vi "AlliGator Python Plugin Plot Data Type.vi"(8 "error in (no error)":errorcluster, 11 "Function Name":string) -> (0 "error out":errorcluster, 3 "Type of Plot Data":T1)   [LabVIEW 2021, in "AlliGator Python Plugins.lvlib"]
doc: "Looks at the python function name to figure out whether it acts on \"All Plots\" or \"Selected Plots\"."
uses:
  AlliGator Python Plugins.lvlib
  AlliGator Type of Plot Data.ctl
panel:
  # "see the AlliGator License on the block diagram (Ctrl+E or Window:Show Block Diagram)"
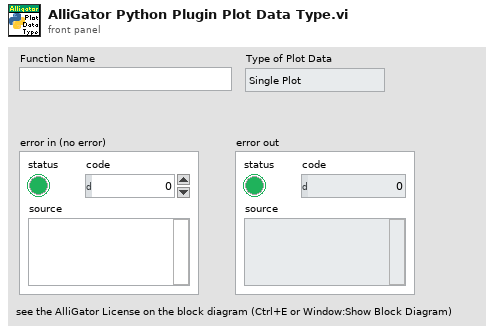
[diagram p1: front panel]
types:
  T1 = typedef "AlliGator Python Plugins.lvlib/AlliGator Type of Plot Data.ctl" = enum16{"Single Plot", "Selected Plots", "All Plots"}
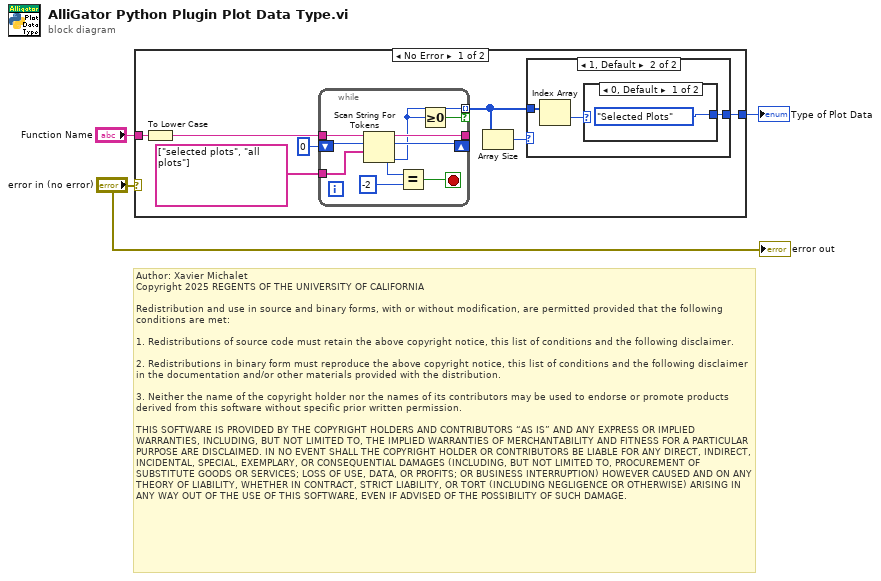
[diagram p0: block diagram]
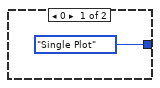
[diagram p2: hidden frame]
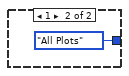
[diagram p3: hidden frame]
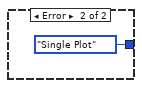
[diagram p4: hidden frame]
diagram:
  # "Author: Xavier Michalet\nCopyright 2025 REGENTS OF THE UNIVERSITY OF CALIFORNIA\n\nRedistribution and use in source and binary forms, with or without modification, are permitted provided that the following conditions are met:\n\n1. Redistributions of source code must retain the above copyright notice, this list of conditions and the following disclaimer.\n\n2. Redistributions in binary form must reproduce the above copyright notice, this list of conditions and the following disclaimer in the documentation and/or other materials provided with the distribution.\n\n3. Neither the name of the copyright holder nor the names of its contributors may be used to endorse or promote products derived from this software without specific prior written permission.\n\nTHIS SOFTWARE IS PROVIDED BY THE COPYRIGHT HOLDERS AND CONTRIBUTORS “AS IS” AND ANY EXPRESS OR IMPLIED WARRANTIES, INCLUDING, BUT NOT LIMITED TO, THE IMPLIED WARRANTIES OF MERCHANTABILITY AND FITNESS FOR A PARTICULAR PURPOSE ARE DISCLAIMED. IN NO EVENT SHALL THE COPYRIGHT HOLDER OR CONTRIBUTORS BE LIABLE FOR ANY DIRECT, INDIRECT, INCIDENTAL, SPECIAL, EXEMPLARY, OR CONSEQUENTIAL DAMAGES (INCLUDING, BUT NOT LIMITED TO, PROCUREMENT OF SUBSTITUTE GOODS OR SERVICES; LOSS OF USE, DATA, OR PROFITS; OR BUSINESS INTERRUPTION) HOWEVER CAUSED AND ON ANY THEORY OF LIABILITY, WHETHER IN CONTRACT, STRICT LIABILITY, OR TORT (INCLUDING NEGLIGENCE OR OTHERWISE) ARISING IN ANY WAY OUT OF THE USE OF THIS SOFTWARE, EVEN IF ADVISED OF THE POSSIBILITY OF SUCH DAMAGE."
  n1 = case shown="No Error" "error in (no error)" {
    tunnel: "Function Name" -> [w10 _]
    tunnel: [w4 AlliGator_Type_of_Plot_Data."Single Plot" ("Type of Plot Data")] -> w2
    frame No Error {
      n2 = To Lower Case(string=w10) -> (all lower case string=w8:string)
      n3 = while {
        tunnel: string[] ["selected plots", "all plots"] -> [w23]
        tunnel: w8 -> [w25]
        tunnel: [w24] -> _
        shift-right: [w21] -> _
        shift-left: 0 ("offset past token") -> [w22]
        tunnel: [w18] -> w6 mode=indexing if=w17
        stop <- w19 stop-if-true
        n4 = Scan String For Tokens(7:w23, 8:w22, 9:w25) -> (0:w18:i32, 2:w21:i32, 3:w24:string)  [unwired: 3 in, 1 out]
        n5 = Equal?(x=w18, y=-2) -> (x = y?=w19:bool)
        n6 = Greater Or Equal To 0?(x=w18) -> (x >= 0?=w17:bool)
      }
      n7 = Array Size(array=w6) -> (size(s)=w5:i32)
      n8 = case shown="1, Default" w5 {
        tunnel: w6 -> [_ w13]
        tunnel: [AlliGator_Type_of_Plot_Data."Single Plot" ("Type of Plot Data") w12] -> w4
        frame 0 {
        }
        frame 1, Default {
          n9 = Index Array(array=w13) -> (element=w14:i32)  [unwired: 1 in]
          n10 = case shown="0, Default" w14 {
            tunnel: [AlliGator_Type_of_Plot_Data."Selected Plots" ("Type of Plot Data") AlliGator_Type_of_Plot_Data."All Plots" ("Type of Plot Data")] -> w12
            frame 0, Default {
            }
            frame 1 {
            }
          }
        }
      }
    }
    frame Error {
    }
  }
  "Type of Plot Data" <- w2
  "error out" <- "error in (no error)"
